vi "TYPEOFPERFUME.vi"() -> (1 "index of element":i32, 2 "Boolean 3":bool, 3 "Boolean 2":bool, 4 "Boolean":bool)   [LabVIEW 2021]
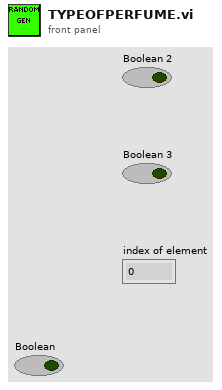
[diagram p1: front panel]
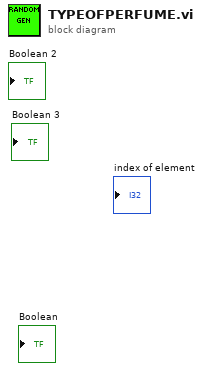
[diagram p0: block diagram]
diagram:
